vi "GetIOWriteStatusMerge.vi"   [LabVIEW 2020]
doc: "Reports the status of written output from the I/O items."
uses:
  <vilib>/eio/EIOGrowableMethodNode/genericMethod/EIOGrowableMethodNode.xnode
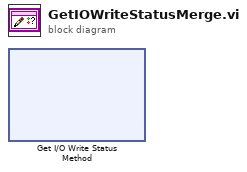
[diagram p0: block diagram]
diagram:
  n1 = xnode "Get I/O Write Status Method"() -> ()  [unwired: 1 in, 4 out]
